vi "OnButton-TimedSequentialPress.vi"(0 "Button":bool, 1 "Timeout (ms)":u32=500, 2 "Press Count":u8=2) -> (3 "Triggered":bool, 4 "Armed":bool, 5 "Timeout":u32, 6 "Remaining":u8)   [LabVIEW 2015]
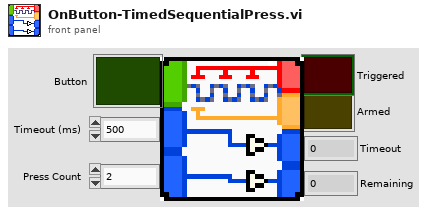
[diagram p1: front panel]
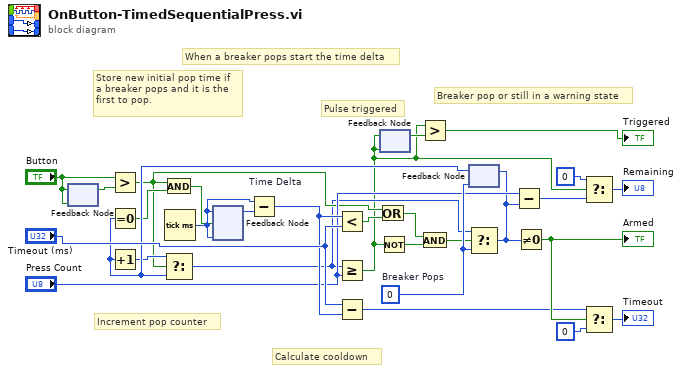
[diagram p0: block diagram]
diagram:
  w20 = u8 0  # Breaker Pops
  # "Pulse triggered"
  # "Breaker pop or still in a warning state"
  # "Calculate cooldown"
  # "Store new initial pop time if\na breaker pops and it is the\nfirst to pop."
  # "Increment pop counter"
  # "When a breaker pops start the time delta"
  n1 = feedback #1("Button") -> (w23:bool)
  n2 = feedback-in #1("Button") -> ()
  n3 = Greater?(x="Button", y=w23) -> (0:w5:bool)
  n4 = Tick Count (ms)() -> (millisecond timer value=w19:u32)
  n5 = feedback #2(w19) -> (w18:u32)
  n6 = Subtract "Time Delta"(x=w19, y=w18) -> (x-y=w16:u32)
  n7 = Less?(x=w16, y="Timeout (ms)") -> (x < y?=w26:bool)
  n8 = Subtract(x="Timeout (ms)", y=w16) -> (x-y=w12:u32)
  n9 = Or(x=w5, y=w26) -> (x .or. y?=w15:bool)
  n10 = feedback #3(w20) -> (w25:u8)
  n11 = Equal To 0?(x=w25) -> (x = 0?=w24:bool)
  n12 = Increment(x=w25) -> (x+1=w21:u8)
  n13 = And(x=w5, y=w24) -> (x .and. y?=w22:bool)
  n14 = Select(t=w21, s=w5, f=w25) -> (s? t:f=w4:u8)
  n15 = feedback-in #2(w19, w22) -> ()
  n16 = Greater Or Equal?(x=w4, y="Press Count") -> (x >= y?=w2:bool)
  n17 = Not(x=w2) -> (.not. x?=w1:bool)
  n18 = feedback-in #4(w2) -> ()
  n19 = feedback #4(w2) -> (w8:bool)
  n20 = Greater?(x=w2, y=w8) -> (0:→"Triggered":bool)
  n21 = And(x=w15, y=w1) -> (x .and. y?=w3:bool)
  n22 = Select(t=w4, s=w3, f=w20) -> (s? t:f=w13:u8)
  n23 = feedback-in #3(w13) -> ()
  n24 = Subtract(x="Press Count", y=w13) -> (x-y=w11:u8)
  n25 = Not Equal To 0?(x=w13) -> (x != 0?=w28:bool)
  "Armed" <- w28
  n26 = Select(t=u8 0, s=w2, f=w11) -> (s? t:f=→"Remaining":u8)
  n27 = Select(t=w12, s=w28, f=u32 0) -> (s? t:f=→"Timeout":u32)
